vi "Cluster to Index.vi"(1 "Object on 8 directions":T1) -> (0 "Index":i32)   [LabVIEW 2021]
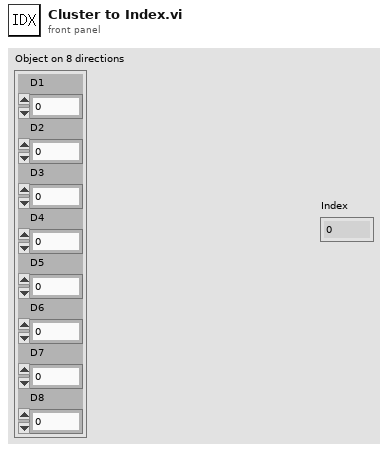
[diagram p1: front panel]
types:
  T1 = cluster{"D1":dbl, "D2":dbl, "D3":dbl, "D4":dbl, "D5":dbl, "D6":dbl, "D7":dbl, "D8":dbl}
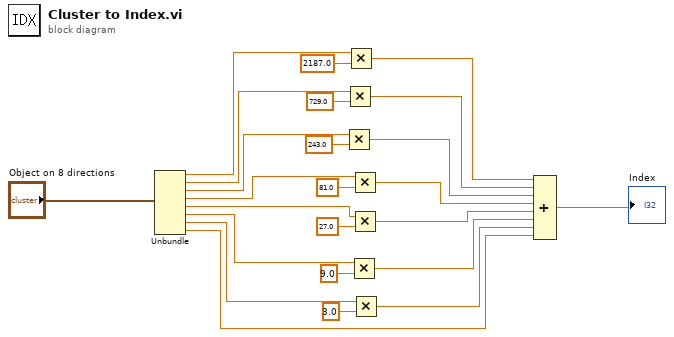
[diagram p0: block diagram]
diagram:
  n1 = Unbundle("Object on 8 directions") -> ("D1"=w1:dbl, "D2"=w2:dbl, "D3"=w3:dbl, "D4"=w4:dbl, "D5"=w5:dbl, "D6"=w6:dbl, "D7"=w7:dbl, "D8"=w21:dbl)
  n2 = Multiply(x=w3, y=243.0) -> (x*y=w10:dbl)
  n3 = Multiply(x=w2, y=729.0) -> (x*y=w9:dbl)
  n4 = Multiply(x=w1, y=2187.0) -> (x*y=w8:dbl)
  n5 = Multiply(x=w6, y=9.0) -> (x*y=w13:dbl)
  n6 = Multiply(x=w4, y=81.0) -> (x*y=w11:dbl)
  n7 = Multiply(x=w5, y=27.0) -> (x*y=w12:dbl)
  n8 = Multiply(x=w7, y=3.0) -> (x*y=w14:dbl)
  n9 = Compound Arithmetic op=ADD(w8, w9, w10, w11, w12, w13, w14, w21) -> (→"Index":dbl)
